vi "Post-Build Action.vi"(5 "Files Generated by Build":path[](array[path]), 6 "Top Level/Always Included VIs":path[](array[path]), 7 "Destination Path":path, 8 "error in (no error)":errorcluster, 9 "Target Name":string, 10 "Build Specification Name":string, 11 "Project Path":path) -> (0 "error out":errorcluster)   [LabVIEW 2023]
uses:
  Capabilities/Capabilities/Utilities/Utilities.lvlib
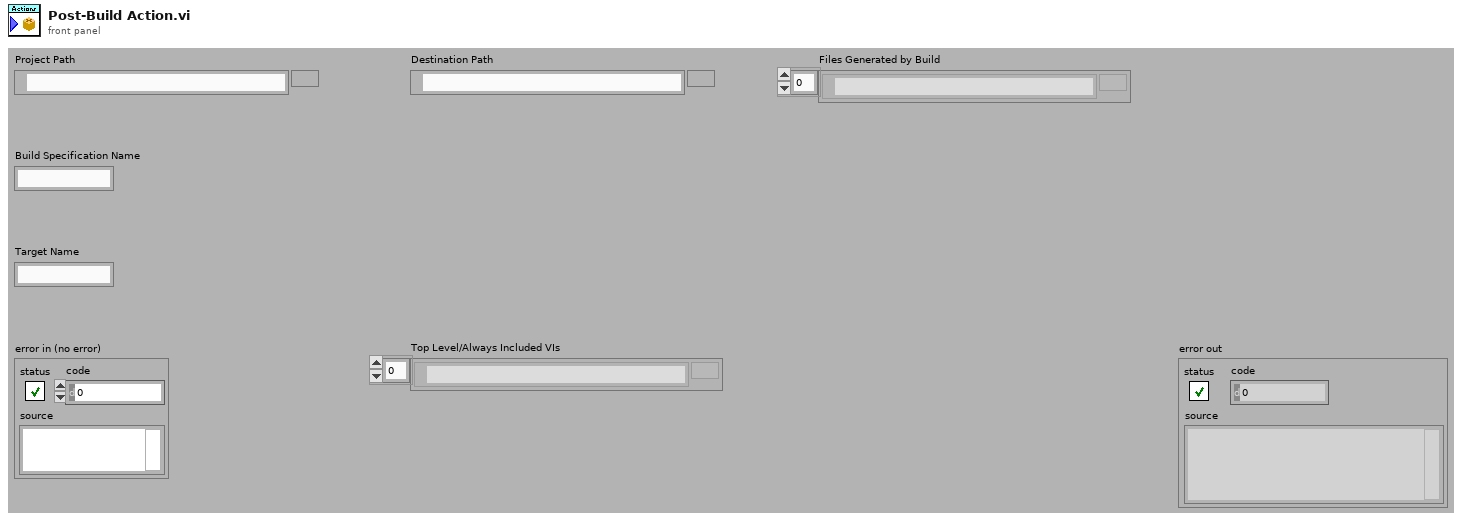
[diagram p1: front panel]
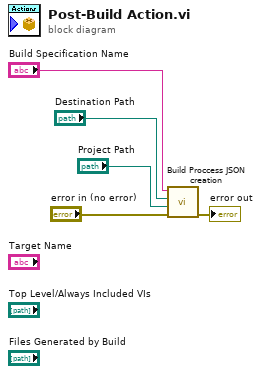
[diagram p0: block diagram]
diagram:
  n1 = call "Build Proccess JSON creation.vi"("error in (no error)"="error in (no error)", "Project Path"="Project Path", "Destination Path"="Destination Path", "Build Specification Name"="Build Specification Name") -> ("error out"=→"error out":errorcluster)  [unwired: 7 in]
